vi "Configure Constant Current.vi"(6 "Voltage Maximum (120.000)":dbl=120.0 min=0.0 max=520.0 step=1.0 format="%.3f", 8 "error in (no error)":errorcluster, 9 "Voltage Minimum (0)":dbl min=0.0 max=520.0 step=1.0 format="%.3f", 10 "CC Current (0)":dbl min=0.0 max=720.0 step=1.0 format="%#.3f", 11 "VISA resource name":refnum<visa-resource-name>) -> (0 "error out":errorcluster, 3 "VISA resource name out":refnum<visa-resource-name>)   [LabVIEW 2020, in "BK Precision 8600 Series.lvlib"]
doc: "Configures the current and voltage max/min limits for constant current (CC) operation."
uses:
  BK Precision 8600 Series.lvlib
panel:
  # "V"
  # "V"
  # "A"
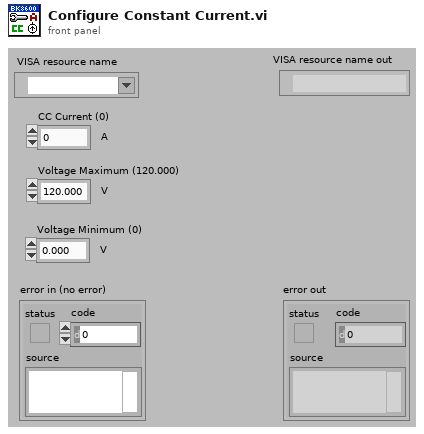
[diagram p1: front panel]
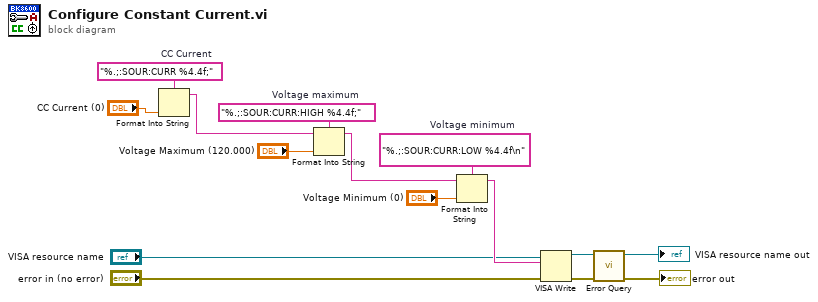
[diagram p0: block diagram]
diagram:
  w8 = "%.;:SOUR:CURR:LOW %4.4f\n"  # Voltage minimum
  w7 = "%.;:SOUR:CURR:HIGH %4.4f;"  # Voltage maximum
  w13 = "%.;:SOUR:CURR %4.4f;"  # CC Current
  n1 = Format Into String(format string=w13, "CC Current (0)") -> (resulting string=w5:string)  [unwired: 2 in, 1 out]
  n2 = Format Into String(format string=w7, initial string=w5, "Voltage Maximum (120.000)") -> (resulting string=w4:string)  [unwired: 1 in, 1 out]
  n3 = Format Into String(format string=w8, initial string=w4, "Voltage Minimum (0)") -> (resulting string=w9:string)  [unwired: 1 in, 1 out]
  n4 = VISA Write(VISA resource name="VISA resource name", write buffer=w9, error in (no error)="error in (no error)") -> (VISA resource name out=w11:refnum<visa-resource-name>, error out=w12:errorcluster)  [unwired: 1 out]
  n5 = call "Error Query.vi"("error in (no error)"=w12, "VISA resource name"=w11) -> ("error out"=→"error out":errorcluster, "VISA resource name out"=→"VISA resource name out":refnum<visa-resource-name>)  [unwired: 6 in, 2 out]
